vi "Nonlinear Calibration Test v5.vi"() -> ()   [LabVIEW 2009]
doc: "This example illustrates the use of a calibration grid to calibrate and correct an image for nonlinear distortion and accurate shape measurements.\n\nThis example loads the image of a calibration grid used to calibrate the system, learns the grid, then loads an image of parts acquired using the same setup. The example then corrects the image in two ways. The first method corrects the entire image and then measures the area of the coins. The second method corrects only the area of the coins and displays the difference in processing time."
uses:
  <vilib>/userDefined/High Color/IMAQdx.ctl
  <vilib>/vision/NI_Vision_Development_Module.lvlib
  <vilib>/vision/driver/NI_Vision_Acquisition_Software.lvlib
panel:
  out "Image 2":T1(plugin-control)
  in  "Camera Name":T2
  in  "Video Modes":i32(listbox)
  in  "stop":bool
  out "Image":T1(plugin-control)
  out "Buffer Number":u32
  out "Frame Rate":dbl(knob) scale=0.0..100.0 scale format="%.1f"
  in  "Red Range":cluster{"Lower value":i32, "Upper value":i32}={"Lower value"=240, "Upper value"=255}
  in  "Green Range":cluster{"Lower value":i32, "Upper value":i32}={"Lower value"=250, "Upper value"=255}
  in  "Blue Range":cluster{"Lower value":i32, "Upper value":i32}={"Lower value"=250, "Upper value"=255}
  in  "Color Mode":u16(ring) items=["RGB", "HSL", "HSV", "HSI"]
  out "Super Filter":T1(plugin-control)
  in  "File Path 2":path=path "C:/Documents and Settings/ekolker/My Documents/OGRE/to be synched/coinMimic2.png"
  in  "Calibration File Path":path
  out "Bottom Image":T1(plugin-control) caption="Calibrated Measurements"
  out "Top Image":T1(plugin-control) caption="Corrected Image"
  # "This step takes measurements in two ways.  The first calculation corrects \nthe entire image, and then takes the measurements.  The second calculation only corrects the coins, and then takes the measurements."
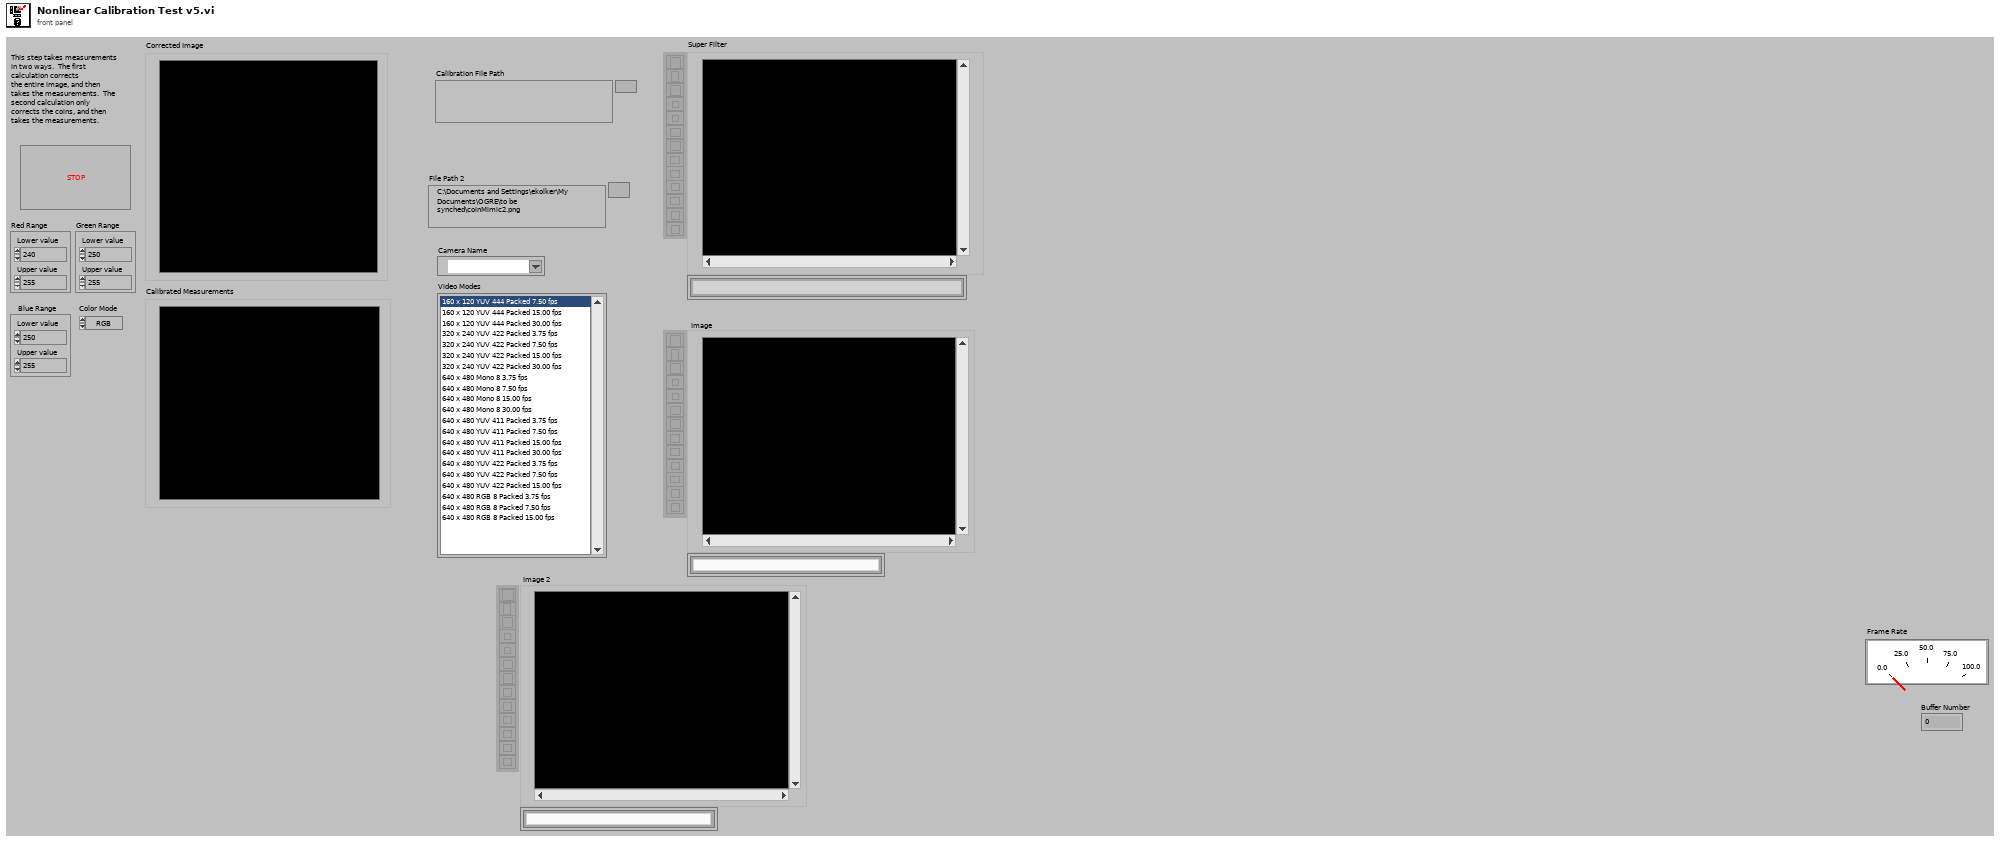
[diagram p1: front panel]
types:
  T1 = typedef "IMAQ Image.ctl" = refnum<image>
  T2 = typedef "IMAQdx.ctl" = refnum<k21>
  T3 = typedef "Image Type" = u32
  T4 = cluster{"X Step":sgl, "Y Step":sgl, "Unit":u32, "Threshold Range":cluster{"Lower value":sgl, "Upper value":sgl}}
  T5 = cluster{"Distortion":u32, "Corrected Image Scaling":u32, "Corrected Image Learn ROI":u32, "Learn Error Map?":bool, "Learn Correction Table?":bool}
  T6 = typedef "Particle Parameters" = i32
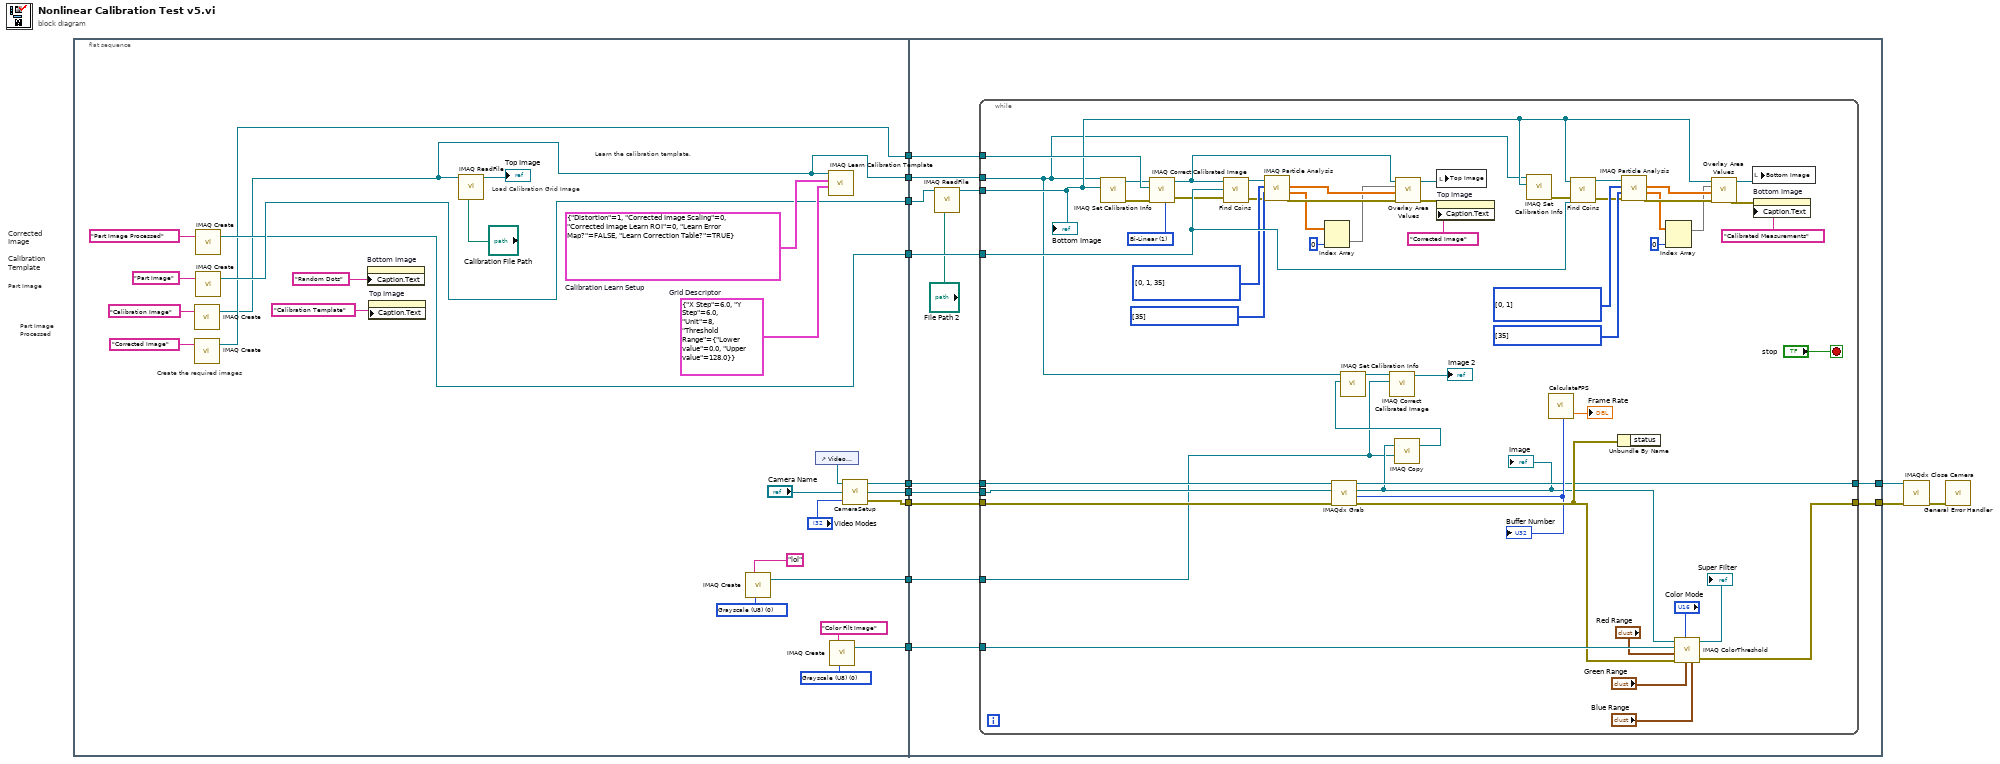
[diagram p0: block diagram]
diagram:
  # "Corrected\nImage"
  # "Part Image Processed"
  # "Calibration Template"
  # "Part Image"
  n1 = flat-sequence {
    tunnel: [w36] -> w12
    tunnel: [w21] -> w11
    tunnel: [w35] -> w10
    tunnel: [w26] -> w9
    tunnel: [w22] -> w5
    tunnel: [w19] -> w4
    tunnel: [w18] -> w3
    tunnel: [w17] -> w2
    tunnel: [w13] -> w1
    tunnel: w12 -> [w47]
    tunnel: w11 -> [w51]
    tunnel: w10 -> [w50]
    tunnel: w9 -> [w49]
    tunnel: [w45] -> w7
    tunnel: [w44] -> w6
    tunnel: w5 -> [w43]
    tunnel: w4 -> [w42]
    tunnel: w3 -> [w41]
    tunnel: w2 -> [w40]
    tunnel: w1 -> [w39]
    frame #0 {
      w15 = T3 0 items=["Grayscale (U8)", "Grayscale (I16)", "Grayscale (SGL)", "Complex (CSG)", "RGB (U32)", "HSL (U32)", "RGB (U64)", "Grayscale (U16)"] ("Image Type")
      w25 = T3 0 items=["Grayscale (U8)", "Grayscale (I16)", "Grayscale (SGL)", "Complex (CSG)", "RGB (U32)", "HSL (U32)", "RGB (U64)", "Grayscale (U16)"] ("Image Type")
      w37 = T4 {"X Step"=6.0, "Y Step"=6.0, "Unit"=8, "Threshold Range"={"Lower value"=0.0, "Upper value"=128.0}}  # Grid Descriptor
      w38 = T5 {"Distortion"=1, "Corrected Image Scaling"=0, "Corrected Image Learn ROI"=0, "Learn Error Map?"=FALSE, "Learn Correction Table?"=TRUE}  # Calibration Learn Setup
      # "Create the required images"
      # "Load Calibration Grid Image"
      # "Learn the calibration template."
      n2 = call "IMAQ Create"("Image Name"="Calibration Image") -> ("New Image"=w21:T1)  [unwired: 3 in, 2 out]
      n3 = call "IMAQ Create"("Image Name"="Corrected Image") -> ("New Image"=w26:T1)  [unwired: 3 in, 2 out]
      n4 = call "IMAQ Create"("Image Name"="Part Image Processed") -> ("New Image"=w35:T1)  [unwired: 3 in, 2 out]
      n5 = call "IMAQ Create"("Image Name"="Part Image") -> ("New Image"=w36:T1)  [unwired: 3 in, 2 out]
      n6 = property on="Bottom Image" class="ImageControl"("Caption.Text"="Random Dots" ("Title")) -> ()  [unwired: 2 in, 2 out]
      n7 = property on="Top Image" class="ImageControl"("Caption.Text"="Calibration Template" ("Title")) -> ()  [unwired: 2 in, 2 out]
      n8 = call "IMAQ ReadFile"("File Path"="Calibration File Path", "Image"=w21) -> ("Image Out"=→"Top Image":T1)  [unwired: 3 in, 6 out]
      n9 = call "IMAQ Create"("Image Name"="lol", "Image Type"=w15) -> ("New Image"=w13:T1)  [unwired: 2 in, 2 out]
      n10 = control-ref of="Video Modes"() -> (w16:refnum<vi>)
      n11 = call "IMAQ Learn Calibration Template"("Grid Descriptor"=w37, "Calibration Learn Setup"=w38, "Image"=w21) -> ()  [unwired: 4 in, 5 out]
      n12 = call "IMAQ Create"("Image Name"="Color Filt Image", "Image Type"=w25) -> ("New Image"=w22:T1)  [unwired: 2 in, 2 out]
      n13 = call "CameraSetup.vi"("Video Modes"="Video Modes", "Camera Name"="Camera Name", "reference"=w16) -> ("error out"=w17:errorcluster, "New Image"=w18:T1, "Session Out"=w19:T2)
    }
    frame #1 {
      n14 = call "IMAQ ReadFile"("File Path"="File Path 2", "Image"=w47) -> ("Image Out"=w46:T1)  [unwired: 3 in, 6 out]
      n15 = while {
        tunnel: w51 -> [w55]
        tunnel: w50 -> [w105]
        tunnel: w49 -> [w93]
        tunnel: w43 -> [w81]
        tunnel: w46 -> [w80]
        tunnel: [w61] -> w45
        tunnel: [w65] -> w44
        tunnel: w42 -> [w60]
        tunnel: w41 -> [w59]
        tunnel: w40 -> [w58]
        tunnel: w39 -> [w53]
        stop <- "stop" stop-if-true
        w85 = u32 1 items=["Zero Order", "Bi-Linear", "Quadratic", "Cubic Spline"] ("Interpolation Type")
        w92 = T6[] [0, 1, 35] items=["Center of Mass X", "Center of Mass Y", "First Pixel X", "First Pixel Y", "Bounding Rect Left", "Bounding Rect Top", "Bounding Rect Right", "Bounding Rect Bottom", "Max Feret Diameter Start X", "Max Feret Diameter Start Y", "Max Feret Diameter End X", "Max Feret Diameter End Y", "Max Horiz. Segment Length Left", "Max Horiz. Segment Length Right", "Max Horiz. Segment Length Row", "-", "Bounding Rect Width", "Bounding Rect Height", "Bounding Rect Diagonal", "Perimeter", "Convex Hull Perimeter", "Holes' Perimeter", "Max Feret Diameter", "Equivalent Ellipse Major Axis", "Equivalent Ellipse Minor Axis", "Equivalent Ellipse Minor Axis (Feret)", "Equivalent Rect Long Side", "Equivalent Rect Short Side", "Equivalent Rect Diagonal", "Equivalent Rect Short Side (Feret)", "Average Horiz. Segment Length", "Average Vert. Segment Length", "Hydraulic Radius", "Waddel Disk Diameter", "-", "Area", "Holes' Area", "Particle & Holes' Area", "Convex Hull Area", "Image Area", "-", "Number of Holes", "Number of Horiz. Segments", "Number of Vert. Segments", "-", "Orientation", "Max Feret Diameter Orientation", "-", "% Area/Image Area", "% Area/(Particle & Holes' Area)", "Ratio of Equivalent Ellipse Axes", "Ratio of Equivalent Rect Sides", "-", "Elongation Factor", "Compactness Factor", "Heywood Circularity Factor", "Type Factor", "-", "Sum X", "Sum Y", "Sum XX", "Sum XY", "Sum YY", "Sum XXX", "Sum XXY", "Sum XYY", "Sum YYY", "-", "Moment of Inertia XX", "Moment of Inertia XY", "Moment of Inertia YY", "Moment of Inertia XXX", "Moment of Inertia XXY", "Moment of Inertia XYY", "Moment of Inertia YYY", "Norm. Moment of Inertia XX", "Norm. Moment of Inertia XY", "Norm. Moment of Inertia YY", "Norm. Moment of Inertia XXX", "Norm. Moment of Inertia XXY", "Norm. Moment of Inertia XYY", "Norm. Moment of Inertia YYY", "Hu Moment 1", "Hu Moment 2", "Hu Moment 3", "Hu Moment 4", "Hu Moment 5", "Hu Moment 6", "Hu Moment 7"] ("Calibrated Measurements")
        w91 = T6[] [35] items=["Center of Mass X", "Center of Mass Y", "First Pixel X", "First Pixel Y", "Bounding Rect Left", "Bounding Rect Top", "Bounding Rect Right", "Bounding Rect Bottom", "Max Feret Diameter Start X", "Max Feret Diameter Start Y", "Max Feret Diameter End X", "Max Feret Diameter End Y", "Max Horiz. Segment Length Left", "Max Horiz. Segment Length Right", "Max Horiz. Segment Length Row", "-", "Bounding Rect Width", "Bounding Rect Height", "Bounding Rect Diagonal", "Perimeter", "Convex Hull Perimeter", "Holes' Perimeter", "Max Feret Diameter", "Equivalent Ellipse Major Axis", "Equivalent Ellipse Minor Axis", "Equivalent Ellipse Minor Axis (Feret)", "Equivalent Rect Long Side", "Equivalent Rect Short Side", "Equivalent Rect Diagonal", "Equivalent Rect Short Side (Feret)", "Average Horiz. Segment Length", "Average Vert. Segment Length", "Hydraulic Radius", "Waddel Disk Diameter", "-", "Area", "Holes' Area", "Particle & Holes' Area", "Convex Hull Area", "Image Area", "-", "Number of Holes", "Number of Horiz. Segments", "Number of Vert. Segments", "-", "Orientation", "Max Feret Diameter Orientation", "-", "% Area/Image Area", "% Area/(Particle & Holes' Area)", "Ratio of Equivalent Ellipse Axes", "Ratio of Equivalent Rect Sides", "-", "Elongation Factor", "Compactness Factor", "Heywood Circularity Factor", "Type Factor", "-", "Sum X", "Sum Y", "Sum XX", "Sum XY", "Sum YY", "Sum XXX", "Sum XXY", "Sum XYY", "Sum YYY", "-", "Moment of Inertia XX", "Moment of Inertia XY", "Moment of Inertia YY", "Moment of Inertia XXX", "Moment of Inertia XXY", "Moment of Inertia XYY", "Moment of Inertia YYY", "Norm. Moment of Inertia XX", "Norm. Moment of Inertia XY", "Norm. Moment of Inertia YY", "Norm. Moment of Inertia XXX", "Norm. Moment of Inertia XXY", "Norm. Moment of Inertia XYY", "Norm. Moment of Inertia YYY", "Hu Moment 1", "Hu Moment 2", "Hu Moment 3", "Hu Moment 4", "Hu Moment 5", "Hu Moment 6", "Hu Moment 7"] ("Pixel Measurements")
        w99 = T6[] [0, 1] items=["Center of Mass X", "Center of Mass Y", "First Pixel X", "First Pixel Y", "Bounding Rect Left", "Bounding Rect Top", "Bounding Rect Right", "Bounding Rect Bottom", "Max Feret Diameter Start X", "Max Feret Diameter Start Y", "Max Feret Diameter End X", "Max Feret Diameter End Y", "Max Horiz. Segment Length Left", "Max Horiz. Segment Length Right", "Max Horiz. Segment Length Row", "-", "Bounding Rect Width", "Bounding Rect Height", "Bounding Rect Diagonal", "Perimeter", "Convex Hull Perimeter", "Holes' Perimeter", "Max Feret Diameter", "Equivalent Ellipse Major Axis", "Equivalent Ellipse Minor Axis", "Equivalent Ellipse Minor Axis (Feret)", "Equivalent Rect Long Side", "Equivalent Rect Short Side", "Equivalent Rect Diagonal", "Equivalent Rect Short Side (Feret)", "Average Horiz. Segment Length", "Average Vert. Segment Length", "Hydraulic Radius", "Waddel Disk Diameter", "-", "Area", "Holes' Area", "Particle & Holes' Area", "Convex Hull Area", "Image Area", "-", "Number of Holes", "Number of Horiz. Segments", "Number of Vert. Segments", "-", "Orientation", "Max Feret Diameter Orientation", "-", "% Area/Image Area", "% Area/(Particle & Holes' Area)", "Ratio of Equivalent Ellipse Axes", "Ratio of Equivalent Rect Sides", "-", "Elongation Factor", "Compactness Factor", "Heywood Circularity Factor", "Type Factor", "-", "Sum X", "Sum Y", "Sum XX", "Sum XY", "Sum YY", "Sum XXX", "Sum XXY", "Sum XYY", "Sum YYY", "-", "Moment of Inertia XX", "Moment of Inertia XY", "Moment of Inertia YY", "Moment of Inertia XXX", "Moment of Inertia XXY", "Moment of Inertia XYY", "Moment of Inertia YYY", "Norm. Moment of Inertia XX", "Norm. Moment of Inertia XY", "Norm. Moment of Inertia YY", "Norm. Moment of Inertia XXX", "Norm. Moment of Inertia XXY", "Norm. Moment of Inertia XYY", "Norm. Moment of Inertia YYY", "Hu Moment 1", "Hu Moment 2", "Hu Moment 3", "Hu Moment 4", "Hu Moment 5", "Hu Moment 6", "Hu Moment 7"] ("Calibrated Measurements")
        w103 = T6[] [35] items=["Center of Mass X", "Center of Mass Y", "First Pixel X", "First Pixel Y", "Bounding Rect Left", "Bounding Rect Top", "Bounding Rect Right", "Bounding Rect Bottom", "Max Feret Diameter Start X", "Max Feret Diameter Start Y", "Max Feret Diameter End X", "Max Feret Diameter End Y", "Max Horiz. Segment Length Left", "Max Horiz. Segment Length Right", "Max Horiz. Segment Length Row", "-", "Bounding Rect Width", "Bounding Rect Height", "Bounding Rect Diagonal", "Perimeter", "Convex Hull Perimeter", "Holes' Perimeter", "Max Feret Diameter", "Equivalent Ellipse Major Axis", "Equivalent Ellipse Minor Axis", "Equivalent Ellipse Minor Axis (Feret)", "Equivalent Rect Long Side", "Equivalent Rect Short Side", "Equivalent Rect Diagonal", "Equivalent Rect Short Side (Feret)", "Average Horiz. Segment Length", "Average Vert. Segment Length", "Hydraulic Radius", "Waddel Disk Diameter", "-", "Area", "Holes' Area", "Particle & Holes' Area", "Convex Hull Area", "Image Area", "-", "Number of Holes", "Number of Horiz. Segments", "Number of Vert. Segments", "-", "Orientation", "Max Feret Diameter Orientation", "-", "% Area/Image Area", "% Area/(Particle & Holes' Area)", "Ratio of Equivalent Ellipse Axes", "Ratio of Equivalent Rect Sides", "-", "Elongation Factor", "Compactness Factor", "Heywood Circularity Factor", "Type Factor", "-", "Sum X", "Sum Y", "Sum XX", "Sum XY", "Sum YY", "Sum XXX", "Sum XXY", "Sum XYY", "Sum YYY", "-", "Moment of Inertia XX", "Moment of Inertia XY", "Moment of Inertia YY", "Moment of Inertia XXX", "Moment of Inertia XXY", "Moment of Inertia XYY", "Moment of Inertia YYY", "Norm. Moment of Inertia XX", "Norm. Moment of Inertia XY", "Norm. Moment of Inertia YY", "Norm. Moment of Inertia XXX", "Norm. Moment of Inertia XXY", "Norm. Moment of Inertia XYY", "Norm. Moment of Inertia YYY", "Hu Moment 1", "Hu Moment 2", "Hu Moment 3", "Hu Moment 4", "Hu Moment 5", "Hu Moment 6", "Hu Moment 7"] ("Pixel Measurements")
        n16 = call "IMAQ Set Calibration Info"("Image Dst"=w80, "Image Src"=w55) -> ("error out"=w78:errorcluster, "Calibrated Image"=w79:T1)  [unwired: 2 in, 6 out]
        n17 = call "IMAQ Correct Calibrated Image"("Interpolation Type"=w85, "error in (no error)"=w78, "Image Dst"=w93, "Image Src"=w79) -> ("error out"=w77:errorcluster, "Corrected Image"=w86:T1)  [unwired: 3 in, 3 out]
        n18 = call "Find Coins.vi"("error in"=w77, "Dest Image"=w105, "Source Image"=w86) -> ("error out"=w76:errorcluster, "Image Out"=w75:T1)  [unwired: 1 out]
        n19 = call "IMAQ Particle Analysis"("error in (no error)"=w76, "Real-World Measurements"=w91, "Pixel Measurements"=w92, "Image"=w75) -> ("error out"=w94:errorcluster, "Particle Measurements (Real-World)"=w88:dbl[][], "Particle Measurements (Pixels)"=w90:dbl[][])  [unwired: 1 in, 4 out]
        n20 = Index Array(array=w88, index (col)=0 ("Index (row)")) -> (element=w89:dbl[])  [unwired: 1 in]
        n21 = call <vilib>:"IMAQdx Grab.vi"("error in"=w58, "Image In"=w59, "Session In"=w60) -> ("error out"=w63:errorcluster, "Buffer Number Out"=w62:u32, "Image Out"=w57:T1, "Session Out"=w61:T2)  [unwired: 1 in, 4 out]
        "Image" <- w57
        "Buffer Number" <- w62
        n22 = call "IMAQ Copy"("Image Dst"=w53, "Image Src"=w57) -> ("Image Dst Out"=w56:T1)  [unwired: 4 in, 1 out]
        n23 = call "IMAQ Set Calibration Info"("Image Dst"=w56, "Image Src"=w55) -> ("Calibrated Image"=w54:T1)  [unwired: 2 in, 7 out]
        n24 = call "IMAQ Correct Calibrated Image"("Image Dst"=w53, "Image Src"=w54) -> ("Corrected Image"=→"Image 2":T1)  [unwired: 5 in, 4 out]
        n25 = call "Overlay Area Values.vi"("error in (no error)"=w94, "Coin Center (X,Y)"=w90, "Measurement Values"=w89, "Image In"=w86) -> ("error out"=w83:errorcluster, "Image Out"=w84:T1)  [unwired: 2 out]
        n26 = local write "Top Image"(w84) -> ()
        n27 = property on="Top Image" class="ImageControl"(error in=w83, "Caption.Text"="Corrected Image" ("Title")) -> ()  [unwired: 1 in, 2 out]
        n28 = call "IMAQ Set Calibration Info"("Image Dst"=w80, "Image Src"=w55) -> ("error out"=w72:errorcluster)  [unwired: 2 in, 7 out]
        n29 = call "CalculateFPS.vi"("buffer number"=w62) -> ("processed FPS"=→"Frame Rate":dbl)  [unwired: 2 out]
        n30 = call "Find Coins.vi"("error in"=w72, "Dest Image"=w105, "Source Image"=w80) -> ("error out"=w74:errorcluster, "Image Out"=w73:T1)  [unwired: 1 out]
        n31 = Unbundle By Name(w63) -> ()  [unwired: 1 out]
        n32 = call "IMAQ Particle Analysis"("error in (no error)"=w74, "Real-World Measurements"=w103, "Pixel Measurements"=w99, "Image"=w73) -> ("error out"=w104:errorcluster, "Particle Measurements (Real-World)"=w101:dbl[][], "Particle Measurements (Pixels)"=w102:dbl[][])  [unwired: 1 in, 4 out]
        n33 = Index Array(array=w101, index (col)=0 ("Index (row)")) -> (element=w98:dbl[])  [unwired: 1 in]
        n34 = call "IMAQ ColorThreshold"("Blue or Luma or Val or Inten Range"="Blue Range", "Green or Sat Range"="Green Range", "Color Mode"="Color Mode", "error in (no error)"=w63, "Red or Hue Range"="Red Range", "Image Dst"=w81, "Image Src"=w57) -> ("error out"=w65:errorcluster, "Image Dst Out"=→"Super Filter":T1)  [unwired: 3 in]
        n35 = call "Overlay Area Values.vi"("error in (no error)"=w104, "Coin Center (X,Y)"=w102, "Measurement Values"=w98, "Image In"=w80) -> ("error out"=w96:errorcluster, "Image Out"=w97:T1)  [unwired: 2 out]
        n36 = local write "Bottom Image"(w97) -> ()
        n37 = property on="Bottom Image" class="ImageControl"(error in=w96, "Caption.Text"="Calibrated Measurements" ("Title")) -> ()  [unwired: 1 in, 2 out]
        "Bottom Image" <- w80
      }
    }
  }
  n38 = call <vilib>:"IMAQdx Close Camera.vi"("error in"=w6, "Session In"=w7) -> ("error out"=w8:errorcluster)  [unwired: 9 out]
  n39 = call <vilib>:"General Error Handler.vi"("error in (no error)"=w8) -> ()  [unwired: 1 in, 14 out]
